vi "CRYUnflatten Test Infor.vi"(10 "Falattend test infor":string) -> (0 "Error?":bool=TRUE, 2 "unflattened test infor data":T1)   [LabVIEW 2013]
uses:
  Typedef Control/CRYStimulus Test Infor Cluster.ctl
panel:
  out "FreqAmpPhase":cluster{"freq":dbl, "ampl":dbl, "cycles":dbl}[](array[cluster]) {"cycles" format="%.2f"; "ampl" format="%.2f"; "freq" format="%.2f"}
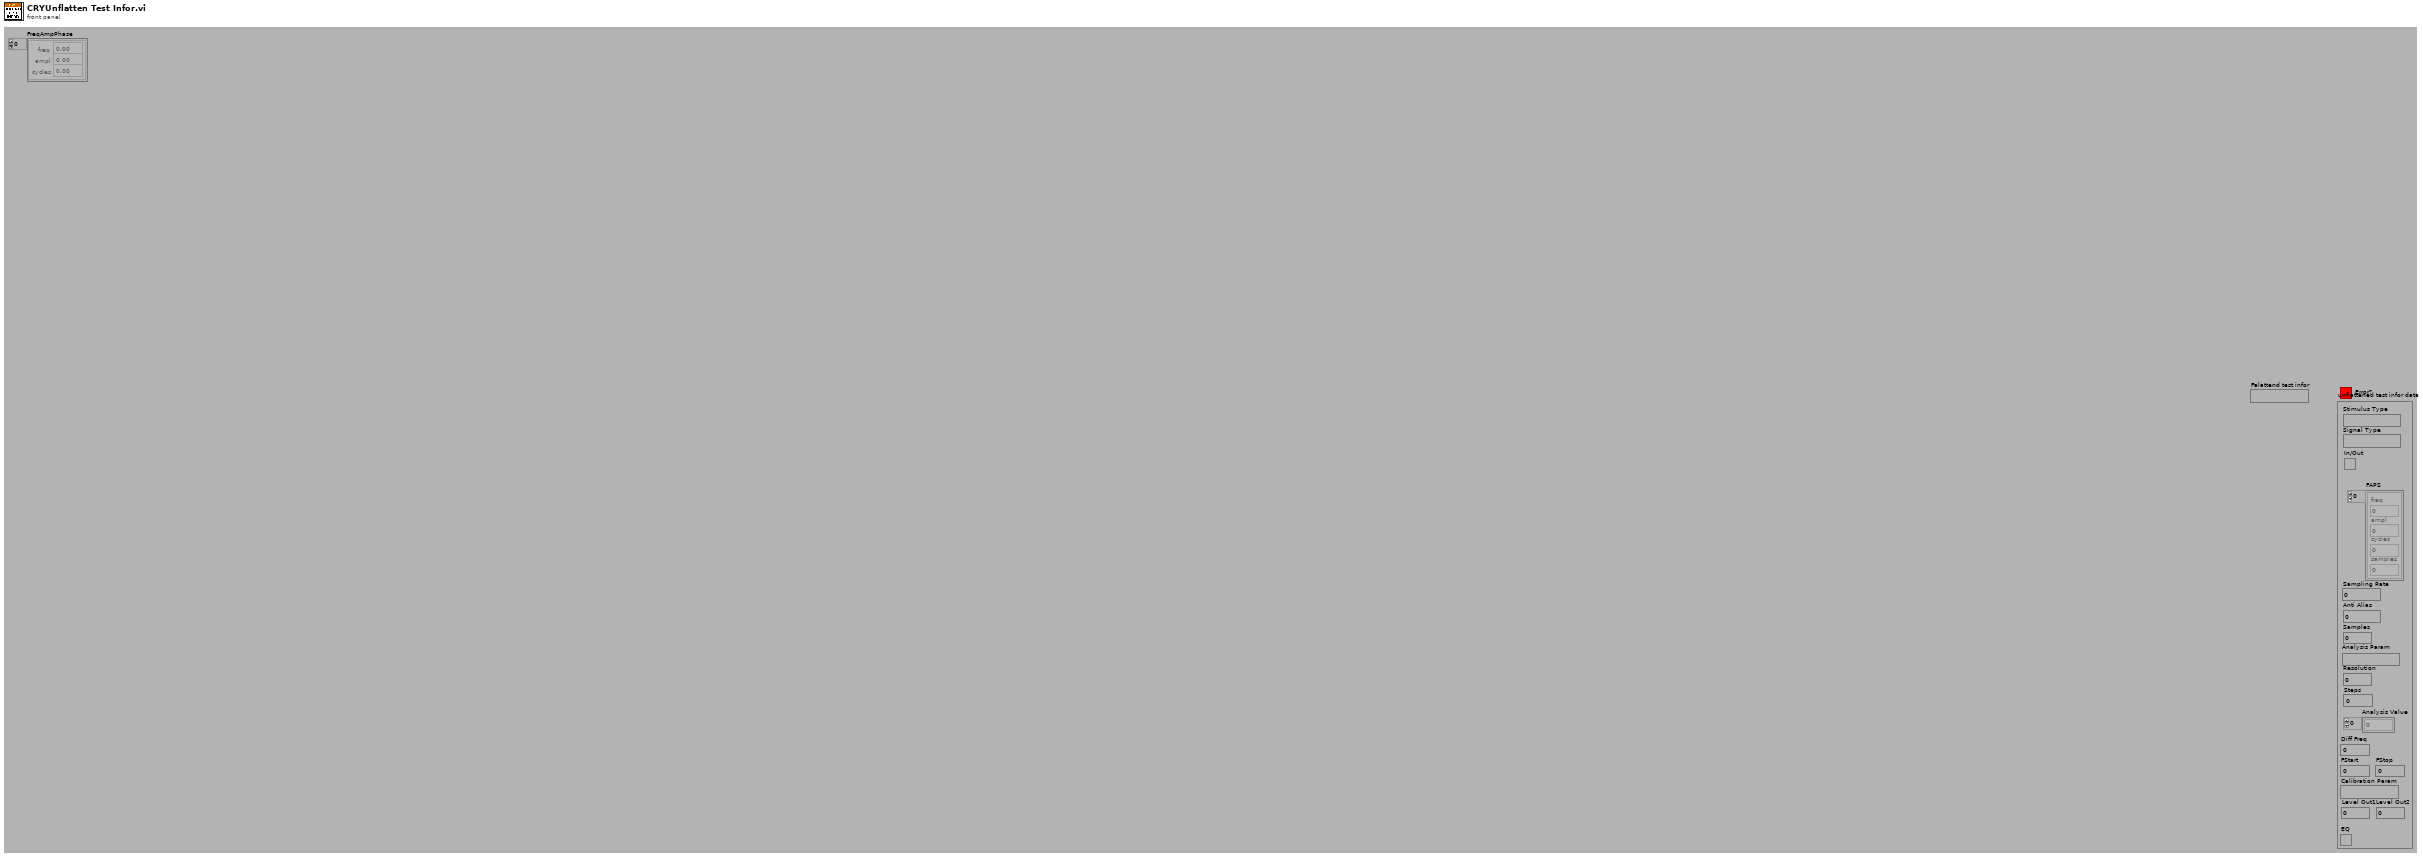
[diagram p1: front panel]
types:
  T1 = typedef "CRYStimulus Test Infor Cluster.ctl" = cluster{"Stimulus Type":string, "Signal Type":string, "In/Out":bool, "FAPS":cluster{"freq":dbl, "ampl":dbl, "cycles":dbl, "samples":i32}[], "Sampling Rate":dbl, "Samples":i32, "Analysis Param":string, "Resolution":u16, "Steps":u32, "Analysis Value":dbl[], "Diff Freq":dbl, "FStart":dbl, "FStop":dbl, "Calibration Param":string, "Anti Alias":dbl, "Level Out1":dbl, "Level Out2":dbl, "EQ":bool}
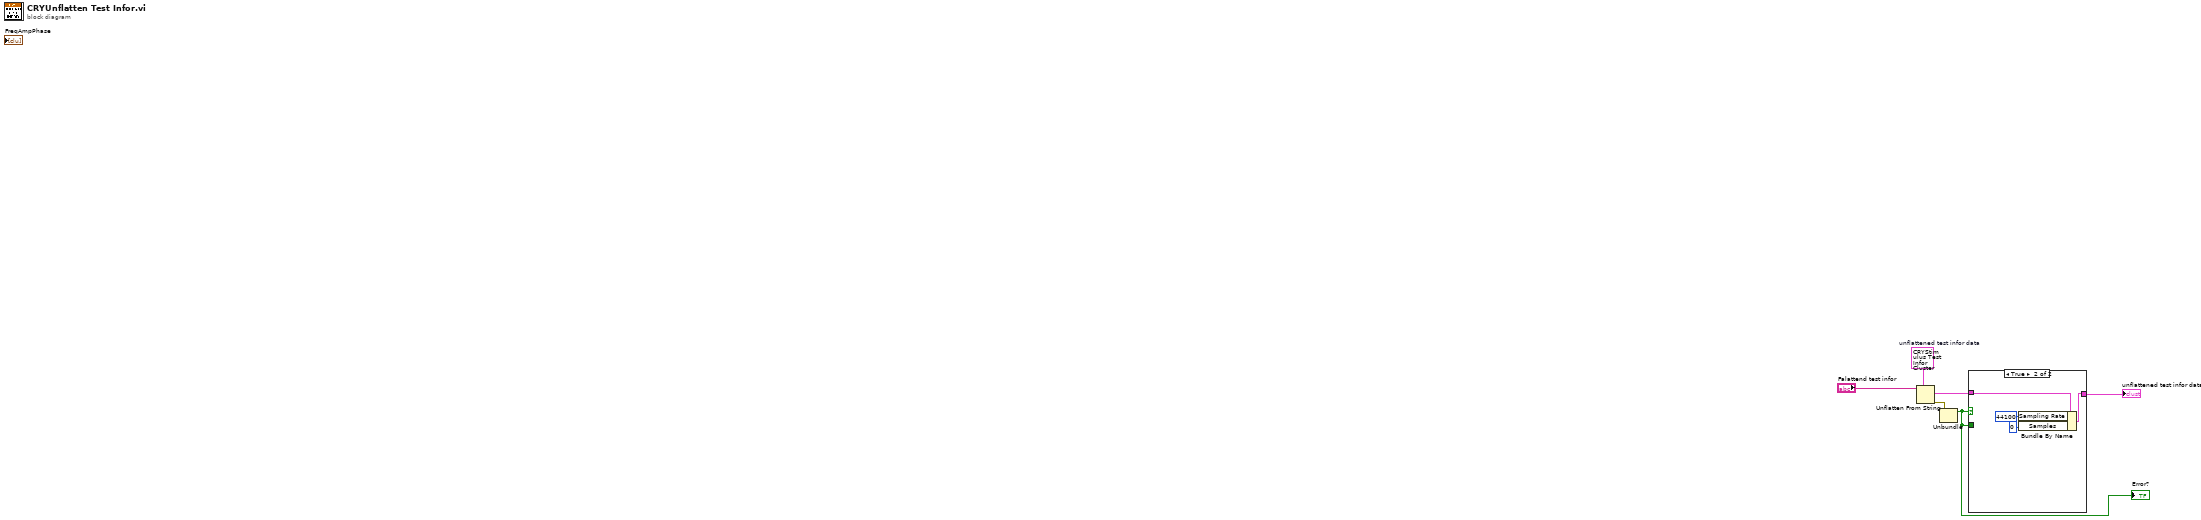
[diagram p0: block diagram]
diagram:
  w2 = T1 {"Stimulus Type"="", "Signal Type"="", "In/Out"=FALSE, "FAPS"=[], "Sampling Rate"=0.0, "Samples"=0, "Analysis Param"="", "Resolution"=0, "Steps"=0, "Analysis Value"=[], "Diff Freq"=0.0, "FStart"=0.0, "FStop"=0.0, "Calibration Param"="", "Anti Alias"=0.0, "Level Out1"=0.0, "Level Out2"=0.0, "EQ"=FALSE}  # unflattened test infor data
  n1 = Unflatten From String(type=w2, binary string="Falattend test infor") -> (value=w3:T1, error out=w5:errorcluster)  [unwired: 1 in, 3 out]
  n2 = Unbundle(w5) -> ("status"=w4:bool)  [unwired: 2 out]
  "Error?" <- w4
  n3 = case shown="True" w4 {
    tunnel: w4 -> [_ _]
    tunnel: w3 -> [w7 w11]
    tunnel: [w7 w10] -> w1
    frame False {
    }
    frame True {
      n4 = Bundle By Name(cluster=w11, "Sampling Rate"=44100, "Samples"=0) -> (w10:T1)
    }
  }
  "unflattened test infor data" <- w1
